vi "SetCurveLength.vi"(8 "error in (no error)":errorcluster caption="错误输入（无错误）", 11 "XYPlot 输入":refnum<class "XYPlot.lvclass">) -> (0 "error out":errorcluster caption="错误输出", 3 "XYPlot 输出":refnum<class "XYPlot.lvclass">)   [LabVIEW 2018, in "DataDisplay.lvlib" / "XYPlot.lvclass"]
uses:
  XYPlot.lvclass
  TypeDefine/DD_Command.ctl
  XYPlot.lvclass/XYPlot.ctl
  DataDisplay.lvlib
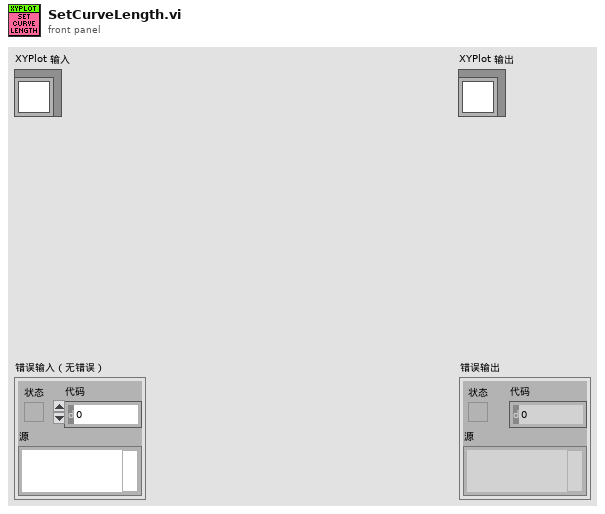
[diagram p1: front panel]
types:
  T1 = typedef "DataDisplay.lvlib/DD_Command.ctl" = cluster{"消息":string, "参数":variant}
  T2 = typedef "DataDisplay.lvlib/DD_CommandQ.ctl" = refnum<queue>
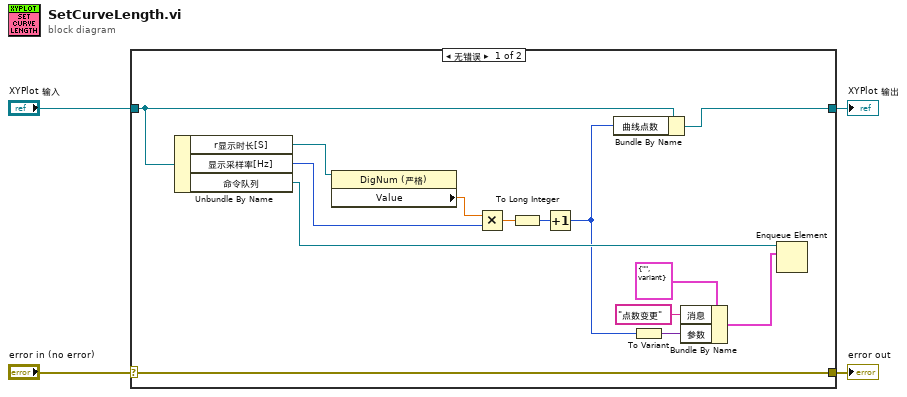
[diagram p0: block diagram]
diagram:
  n1 = case shown="无错误" "error in (no error)" {
    selector: "error in (no error)" -> [w18 w20]
    tunnel: [w18 w20] -> w3
    tunnel: [w11 w19] -> w1
    tunnel: "XYPlot 输入" -> [w17 w19]
    frame No Error {
      n2 = Unbundle By Name(w17) -> ("r显示时长[S]"=w13:refnum<vi>, "显示采样率[Hz]"=w14:i32, "命令队列"=w10:T2)
      n3 = property class="DigNum (严格)"(reference=w13) -> ("Value"=w16:dbl)  [unwired: 1 in, 2 out]
      n4 = Multiply(x=w16, y=w14) -> (x*y=w15:dbl)
      n5 = To Long Integer(number=w15) -> (32bit integer=w12:i32)
      n6 = Increment(x=w12) -> (x+1=w6:i32)
      n7 = Bundle By Name(cluster=w17, "曲线点数"=w6) -> (w11:refnum<class "XYPlot.lvclass">)
      n8 = To Variant(anything=w6) -> (Variant=w5:variant)
      n9 = Bundle By Name(cluster=T1 {"消息"="", "参数"=variant} ("命令"), "消息"="点数变更", "参数"=w5) -> (w7:T1)
      n10 = Enqueue Element(queue=w10, element=w7) -> ()  [unwired: 2 in, 3 out]
    }
    frame Error {
    }
  }
  "error out" <- w3
  "XYPlot 输出" <- w1
